vi "2.4a.vi"() -> ()   [LabVIEW 2020]
panel:
  out "output array":string[](array[string])
  in  "Array":string[][](array[string])
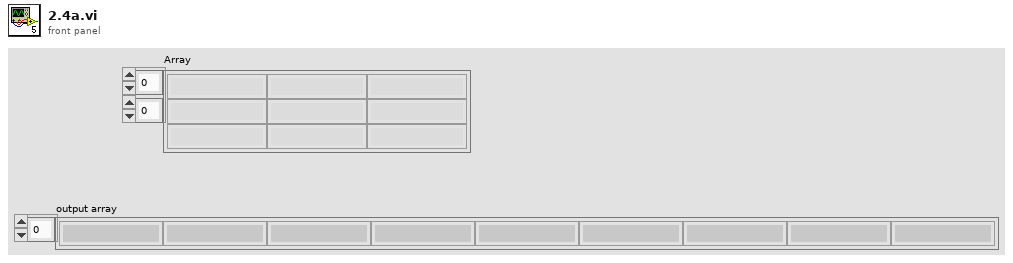
[diagram p1: front panel]
types:
  T1 = enum16{"open", "replace", "create", "open or create", "replace or create", "replace or create with confirmation"}
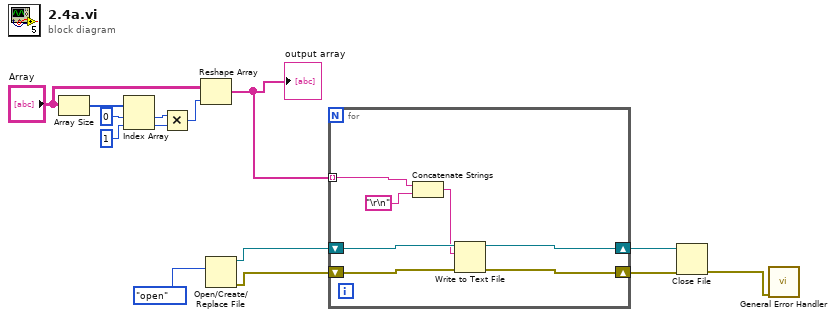
[diagram p0: block diagram]
diagram:
  n1 = Array Size(array="Array") -> (size(s)=w13:i32[])
  n2 = Index Array(array=w13, index #1=0 ("index"), index #2=1 ("index")) -> (element #1=w12:i32, element #2=w11:i32)
  n3 = Multiply(x=w12, y=w11) -> (x*y=w8:i32)
  n4 = Reshape Array("Array", w8) -> (w4:string[])
  "output array" <- w4
  n5 = Open/Create/Replace File(operation (0:open)=T1."open") -> (refnum out=w6:refnum<file>, error out=w5:errorcluster)  [unwired: 5 in, 1 out]
  n6 = for {
    tunnel: w4 -> [w17] mode=indexing
    shift-right: [w19] -> w3
    shift-left: w6 -> [w21]
    shift-right: [w18] -> w2
    shift-left: w5 -> [w20]
    n7 = Concatenate Strings(w17, "\r\n") -> (w15:string)
    n8 = Write to Text File(file (use dialog)=w21, text=w15, error in=w20) -> (refnum out=w19:refnum<file>, error out=w18:errorcluster)  [unwired: 1 in, 1 out]
  }
  n9 = Close File(refnum=w3, error in=w2) -> (error out=w1:errorcluster)  [unwired: 1 out]
  n10 = call <vilib>:"General Error Handler.vi"("error in (no error)"=w1) -> ()  [unwired: 10 in, 5 out]
